vi "Distortions.vi"   [LabVIEW 2013]
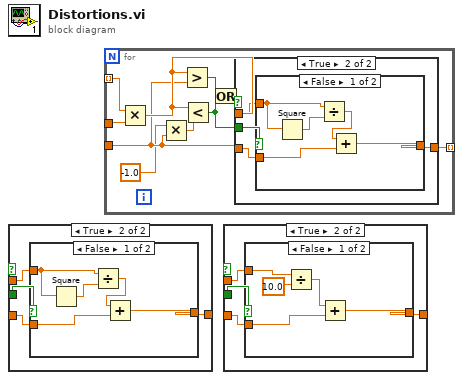
[diagram p0: block diagram]
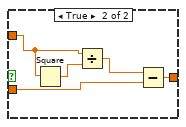
[diagram p3: hidden frame]
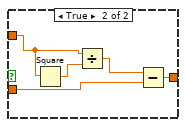
[diagram p5: hidden frame]
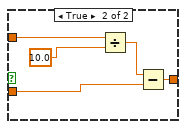
[diagram p7: hidden frame]
diagram:
  n1 = case shown="True" {
    selector: _ -> [_ _]
    tunnel: _ -> [w1 w2]
    tunnel: [w1 w3] -> _
    tunnel: _ -> [_ w4]
    tunnel: _ -> [_ w5]
    frame False {
    }
    frame True {
      n2 = case shown="False" w5 {
        tunnel: w4 -> [w10 w15]
        tunnel: [w9 w14] -> w3
        tunnel: w2 -> [w7 w12]
        frame False {
          n3 = Square(x=w7) -> (x^2=w8:dbl)
          n4 = Divide(x=w7, y=w8) -> (x/y=w6:dbl)
          n5 = Add(x=w6, y=w10) -> (x+y=w9:dbl)
        }
        frame True {
          n6 = Square(x=w12) -> (x^2=w13:dbl)
          n7 = Divide(x=w12, y=w13) -> (x/y=w11:dbl)
          n8 = Subtract(x=w11, y=w15) -> (x-y=w14:dbl)
        }
      }
    }
  }
  n9 = for {
    tunnel: _ -> [w23] mode=indexing
    tunnel: _ -> [w24]
    tunnel: [w25] -> _ mode=indexing
    tunnel: _ -> [w17]
    n10 = Multiply(x=w23, y=w24) -> (x*y=w20:dbl)
    n11 = Multiply(x=-1.0, y=w17) -> (x*y=w18:dbl)
    n12 = Greater?(x=w20, y=w17) -> (0:w22:bool)
    n13 = Less?(x=w20, y=w18) -> (x < y?=w19:bool)
    n14 = Or(x=w22, y=w19) -> (x .or. y?=w21:bool)
    n15 = case shown="True" w21 {
      tunnel: w20 -> [w26 w27]
      tunnel: [w26 w28] -> w25
      tunnel: w17 -> [_ w29]
      tunnel: w19 -> [_ w30]
      frame False {
      }
      frame True {
        n16 = case shown="False" w30 {
          tunnel: w29 -> [w35 w40]
          tunnel: [w34 w39] -> w28
          tunnel: w27 -> [w32 w37]
          frame False {
            n17 = Square(x=w32) -> (x^2=w33:dbl)
            n18 = Divide(x=w32, y=w33) -> (x/y=w31:dbl)
            n19 = Add(x=w31, y=w35) -> (x+y=w34:dbl)
          }
          frame True {
            n20 = Square(x=w37) -> (x^2=w38:dbl)
            n21 = Divide(x=w37, y=w38) -> (x/y=w36:dbl)
            n22 = Subtract(x=w36, y=w40) -> (x-y=w39:dbl)
          }
        }
      }
    }
  }
  n23 = case shown="True" {
    selector: _ -> [_ _]
    tunnel: _ -> [w41 w42]
    tunnel: [w41 w43] -> _
    tunnel: _ -> [_ w44]
    tunnel: _ -> [_ w45]
    frame False {
    }
    frame True {
      n24 = case shown="False" w45 {
        tunnel: w44 -> [w47 w52]
        tunnel: [w46 w51] -> w43
        tunnel: w42 -> [w49 w54]
        frame False {
          n25 = Divide(x=w49, y=10.0) -> (x/y=w48:dbl)
          n26 = Add(x=w48, y=w47) -> (x+y=w46:dbl)
        }
        frame True {
          n27 = Divide(x=w54, y=10.0) -> (x/y=w53:dbl)
          n28 = Subtract(x=w53, y=w52) -> (x-y=w51:dbl)
        }
      }
    }
  }
